vi "Test get item at grid point.vi"(11 "Test Case In":refnum<class "Test Cases.lvclass">) -> (0 "error out":errorcluster, 3 "Test Case Out":refnum<class "Test Cases.lvclass">)   [LabVIEW 2023, in "Test Cases.lvclass"]
uses:
  Test Cases.lvclass
  C:/Program Files/National Instruments/LabVIEW 2025/vi.lib/Astemes/LUnit/Test Case.lvclass
  source/Grid/SourceGrid.lvclass
  source/Cells/Cell/Cell.lvclass
  <vilib>/Astemes/LUnit/Test Case.lvclass/Test Case.ctl
  Test Cases.lvclass/Test Cases.ctl
  <vilib>/Astemes/LUnit/Test Case.lvclass
  D:/git/Sourcegrid-LabVIEW/dll/SourceGrid.dll
  dll/SourceGrid.dll
panel:
  in  "stop":bool
  in  "Grid Container":refnum<k24>(container)
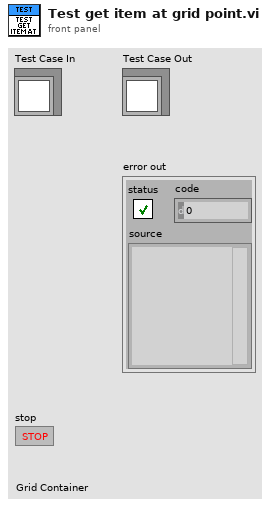
[diagram p1: front panel]
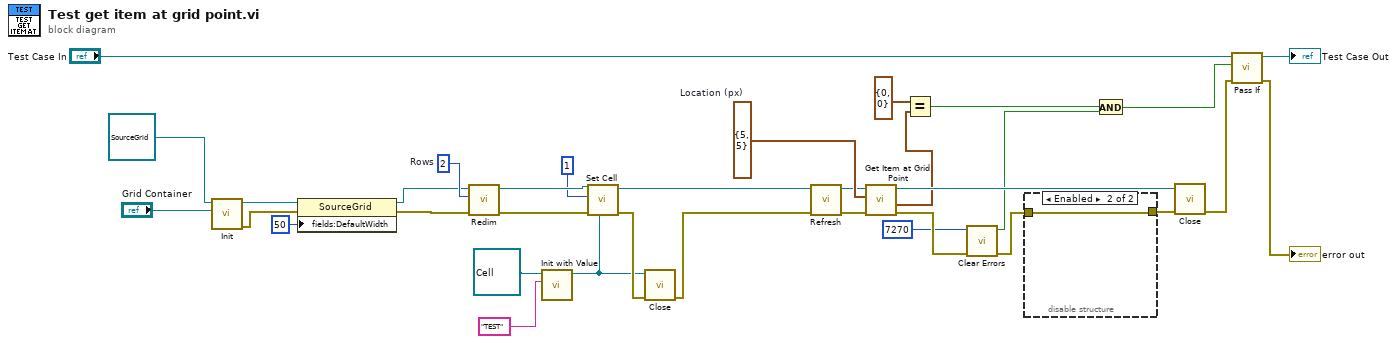
[diagram p0: block diagram]
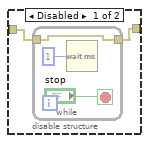
[diagram p2: hidden frame]
diagram:
  w19 = cluster{"X":i32, "Y":i32} {"X"=5, "Y"=5}  # Location (px)
  w31 = 2  # Rows
  n1 = call-dynamic "Init.vi"("Sourcegrid Container"="Grid Container", "Grid in"=refnum<class "SourceGrid.lvclass"> refnum) -> ("error out"=w21:errorcluster, "Grid out"=w28:refnum<class "SourceGrid.lvclass">)  [unwired: 8 in]
  n2 = property class="SourceGrid"(reference=w28, error in=w21, "fields:DefaultWidth"=50 ("DefaultWidth")) -> (reference out=w27:refnum<class "SourceGrid.lvclass">, error out=w26:errorcluster)
  n3 = call "Redim.vi"("error in"=w26, "Rows"=w31, "Sourcegrid in"=w27) -> ("error out"=w18:errorcluster, "Sourcegrid out"=w24:refnum<class "SourceGrid.lvclass">)  [unwired: 7 in]
  n4 = call-dynamic "Init with Value.vi"("Value"="TEST", "Cell in"=refnum<class "Cell.lvclass"> refnum) -> ("Cell out"=w8:refnum<class "Cell.lvclass">)  [unwired: 8 in, 1 out]
  n5 = call "Set Cell.vi"("Cell"=w8, "error in"=w18, "Row"=1, "Sourcegrid in"=w24) -> ("error out"=w10:errorcluster, "Sourcegrid out"=w16:refnum<class "SourceGrid.lvclass">)  [unwired: 6 in]
  n6 = call-dynamic "Close.vi"("error in"=w10, "Cell in"=w8) -> ("error out"=w9:errorcluster)  [unwired: 8 in, 1 out]
  n7 = call "Refresh.vi"("error in"=w9, "SourceGrid in"=w16) -> ("error out"=w17:errorcluster, "SourceGrid out"=w15:refnum<class "SourceGrid.lvclass">)  [unwired: 8 in]
  n8 = call "Get Item at Grid Point.vi"("error in"=w17, "Location"=w19, "SourceGrid in"=w15) -> ("error out"=w14:errorcluster, "Cell Position"=w7:cluster{"Row":i32, "Column":i32}, "SourceGrid out"=w22:refnum<class "SourceGrid.lvclass">)  [unwired: 5 in, 1 out]
  n9 = Equal?(x=cluster{"Row":i32, "Column":i32} {"Row"=0, "Column"=0}, y=w7) -> (x = y?=w5:bool)
  n10 = call <vilib>:"Clear Errors.vi"("error in (no error)"=w14, "specific error code to clear (0: all)"=7270) -> ("error out"=w4:errorcluster, "specific error cleared?"=w2:bool)  [unwired: 4 in]
  n11 = disable-structure shown="Enabled" {
    disable-tunnel: w4 -> [w36 w40]
    disable-tunnel: [w35 w40] -> w20
    frame Disabled {
      n12 = while {
        tunnel: w36 -> [w37]
        tunnel: [w37] -> w35
        stop <- "stop" stop-if-true
        n13 = Wait (ms)(milliseconds to wait=u32 1) -> ()  [unwired: 1 out]
      }
    }
    frame Enabled {
    }
  }
  n14 = And(x=w5, y=w2) -> (x .and. y?=w1:bool)
  n15 = call-dynamic "Close.vi"("error in"=w20, "Sourcegrid in"=w22) -> ("error out"=w30:errorcluster)  [unwired: 8 in, 1 out]
  n16 = call <vilib>:"Pass If.vi"("error in (no error)"=w30, "Pass?"=w1, "LUnit Test Case In"="Test Case In") -> ("error out"=→"error out":errorcluster, "LUnit Test Case Out"=→"Test Case Out":refnum<class "Test Cases.lvclass">)  [unwired: 7 in]
